vi "SetLowerBound.vi"(8 "error in":errorcluster, 10 "LowerBound":dbl, 11 "RealMeasureLimit in":refnum<class "RealMeasureLimit.lvclass">) -> (0 "error out":errorcluster, 3 "RealMeasureLimit out":refnum<class "RealMeasureLimit.lvclass">)   [LabVIEW 2021, in "ProligentXMLGenerator.lvlib" / "RealMeasureLimit.lvclass"]
doc: "Real Measure Limit Lower Bound"
uses:
  RealMeasureLimit.lvclass
  RealMeasureLimit.lvclass/RealMeasureLimit.ctl
  RangeMeasureLimit/RangeMeasureLimit.lvclass
  Base/Decimal/Decimal.lvclass
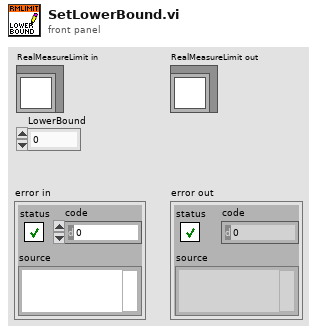
[diagram p1: front panel]
types:
  T1 = typedef "ProligentXMLGenerator.lvlib/RealMeasureLimit.lvclass/Data.ctl" = cluster{"LowerBound":refnum<class "Decimal.lvclass">, "HigherBound":refnum<class "Decimal.lvclass">}
  T2 = typedef "ProligentXMLGenerator.lvlib/RangeMeasureLimit.lvclass/ComparisonType.ctl" = enum16{"LowerBound <= X <= HigherBound", "LowerBound < X <= HigherBound", "LowerBound <= X < HigherBound", "LowerBound < X < HigherBound", "LowerBound <= X", "LowerBound < X", "X <= HigherBound", "X < HigherBound", "X == HigherBound", "X != HigherBound", "X <= LowerBound OR HigherBound <= X", "X < LowerBound OR HigherBound <= X", "X <= LowerBound OR HigherBound < X", "X < LowerBound OR HigherBound < X"}
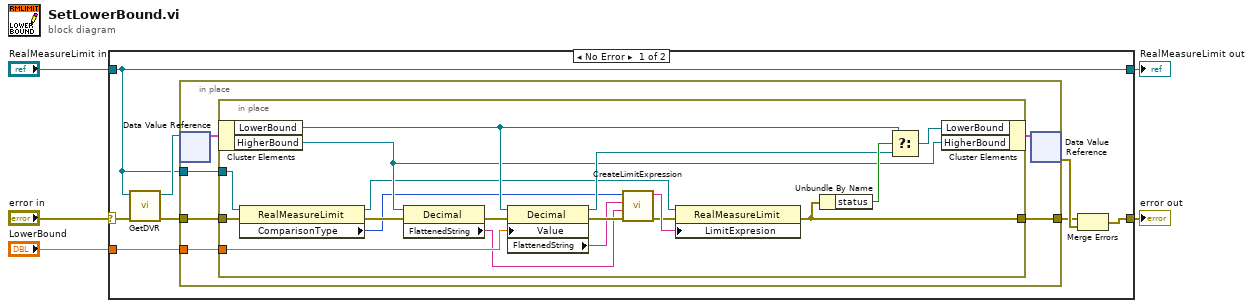
[diagram p0: block diagram]
diagram:
  n1 = case shown="No Error" "error in" {
    selector: "error in" -> [w7 w38]
    tunnel: "RealMeasureLimit in" -> [w6 w39]
    tunnel: [w12 w38] -> w2
    tunnel: "LowerBound" -> [w11 _]
    tunnel: [w6 w39] -> w1
    frame No Error {
      n2 = call "GetDVR.vi"("error in"=w7, "RealMeasureLimit"=w6) -> ("error out"=w10:errorcluster, "DVRReference"=w13:refnum<data-value>)  [unwired: 8 in]
      n3 = in-place "In Place Element Structure" {
        in-place-border: w11 -> [w19]
        in-place-border: w10 -> [w16]
        in-place-border: [w15] -> w8
        in-place-border: w6 -> [w14]
        n4 = in-place-dvr #1(w13) -> (w18:T1)  [unwired: 1 out]
        n5 = in-place "In Place Element Structure" {
          in-place-border: w19 -> [w32]
          in-place-border: w16 -> [w23]
          in-place-border: [w35] -> w15
          in-place-border: w14 -> [w24]
          n6 = in-place-cluster #2(w18) -> ("LowerBound"=w29:refnum<class "Decimal.lvclass">, "HigherBound"=w25:refnum<class "Decimal.lvclass">)
          n7 = property class="RealMeasureLimit"(reference=w24, error in=w23) -> (reference out=w22:refnum<class "RealMeasureLimit.lvclass">, error out=w21:errorcluster, "ComparisonType"=w20:T2)
          n8 = property class="Decimal"(reference=w25, error in=w21) -> (error out=w34:errorcluster, "FlattenedString"=w31:string)  [unwired: 1 out]
          n9 = property class="Decimal"(reference=w29, error in=w34, "Value"=w32) -> (reference out=w26:refnum<class "Decimal.lvclass">, error out=w33:errorcluster, "FlattenedString"=w30:string)
          n10 = call "CreateLimitExpression.vi"("error in"=w33, "HigherBound"=w31, "LowerBound"=w30, "ComparisonType"=w20) -> ("error out"=w36:errorcluster, "LimitExpression"=w37:string)  [unwired: 6 in]
          n11 = property class="RealMeasureLimit"(reference=w22, error in=w36, "LimitExpresion"=w37) -> (error out=w35:errorcluster)  [unwired: 1 out]
          n12 = Unbundle By Name(w35) -> ("status"=w27:bool)
          n13 = Select(t=w29, s=w27, f=w26) -> (s? t:f=w28:refnum<class "Decimal.lvclass">)
          n14 = in-place-cluster #2("LowerBound"=w28, "HigherBound"=w25) -> (w17:T1)
        }
        n15 = in-place-dvr #1(w17) -> (w9:errorcluster)  [unwired: 1 out]
      }
      n16 = Merge Errors(w8, w9) -> (w12:errorcluster)
    }
    frame Error {
    }
  }
  "error out" <- w2
  "RealMeasureLimit out" <- w1
